vi "Beta CDF.vi"(9 "b":dbl=4.0, 10 "a":dbl=2.0, 11 "x":dbl=0.5) -> (0 "error":i32, 3 "cdf(x)":dbl=0.8125)   [LabVIEW 2020, in "NI_Gmath.lvlib"]
doc: "Computes the continuous cumulative distribution function (CDF), or the probability that the random variate X, where X describes the selected distribution type, has a value less than or equal to <B>x</B>. You must manually select the polymorphic instance to use."
uses:
  <vilib>/gmath/NI_Gmath.lvlib
  <vilib>/gmath/statdist.llb/st_error_code.ctl
  <vilib>/gmath/SpecialFunctions.llb/Incomplete Beta Function.vi
panel:
  # "Beta CDF"
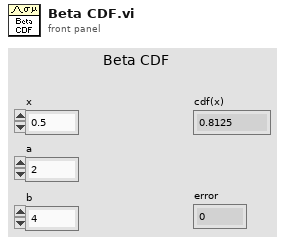
[diagram p1: front panel]
types:
  T1 = typedef "NI_Gmath.lvlib/st_error_code.ctl" = i32
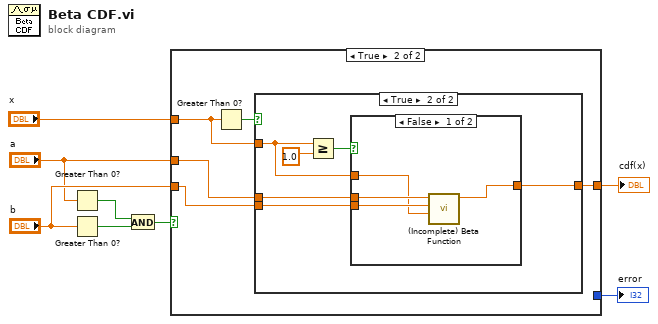
[diagram p0: block diagram]
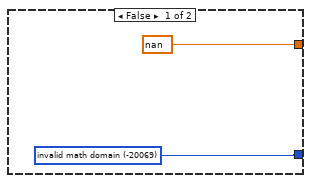
[diagram p2: hidden frame]
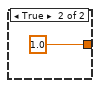
[diagram p4: hidden frame]
diagram:
  n1 = Greater Than 0?(x="a") -> (x > 0?=w1:bool)
  n2 = Greater Than 0?(x="b") -> (x > 0?=w2:bool)
  n3 = And(x=w1, y=w2) -> (x .and. y?=w3:bool)
  n4 = case shown="True" w3 {
    tunnel: "b" -> [_ w11]
    tunnel: [w9 _] -> w8
    tunnel: [nan w14] -> w7
    tunnel: "x" -> [_ w13]
    tunnel: "a" -> [_ w12]
    frame False {
      w9 = T1 -20069 items=["invalid math domain"=-20069, "Fourier interpolation size m >= n"=-20070, "empty array"=-20003] ("stat interp error code")
    }
    frame True {
      n5 = Greater Than 0?(x=w13) -> (x > 0?=w15:bool)
      n6 = case shown="True" w15 {
        tunnel: [_ w19] -> w14
        tunnel: w13 -> [_ w16]
        tunnel: w12 -> [_ w18]
        tunnel: w11 -> [_ w17]
        frame False {
        }
        frame True {
          n7 = Greater Or Equal?(x=w16, y=1.0) -> (x >= y?=w20:bool)
          n8 = case shown="False" w20 {
            tunnel: [w25 1.0] -> w19
            tunnel: w18 -> [w24 _]
            tunnel: w17 -> [w23 _]
            tunnel: w16 -> [w22 _]
            frame False {
              n9 = call-poly <vilib>:"(Incomplete) Beta Function.vi"("a"=w22, "y"=w23, "x"=w24) -> ("b(x, y, a)"=w25:dbl)  [unwired: 8 in]
            }
            frame True {
            }
          }
        }
      }
    }
  }
  "cdf(x)" <- w7
  "error" <- w8
